vi "testMostCommon.vi"   [LabVIEW 2017]
uses:
  <vilib>/addons/_JKI Toolkits/Caraya/classes/Assert/Assert Equal Value_Variant.vi
  <vilib>/addons/_JKI Toolkits/Caraya/classes/Assert/Assert.lvclass
  <vilib>/addons/_JKI Toolkits/Caraya/classes/Test/Test.lvclass
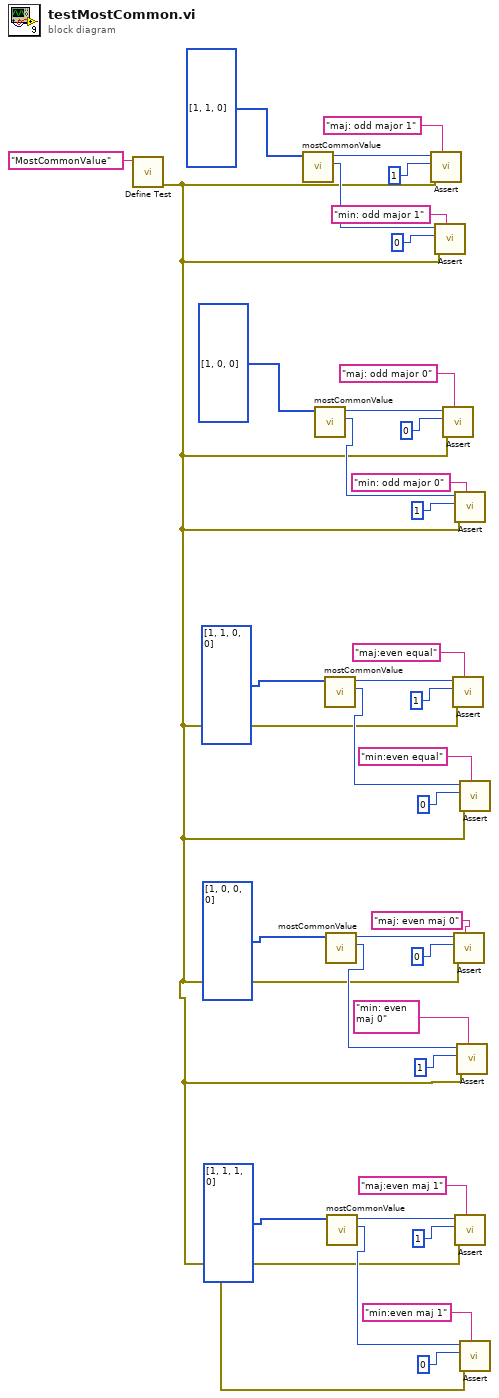
[diagram p0: block diagram]
diagram:
  n1 = call <vilib>:"Define Test.vi"("Label (VI Title)"="MostCommonValue") -> ("error out"=w1:errorcluster)  [unwired: 10 in]
  n2 = call "mostCommonValue.vi"("Array"=i32[] [1, 1, 0]) -> ("Minor"=w16:i32, "Major"=w36:i32)  [unwired: 9 in]
  n3 = call "mostCommonValue.vi"("Array"=i32[] [1, 0, 0]) -> ("Minor"=w11:i32, "Major"=w33:i32)  [unwired: 9 in]
  n4 = call "mostCommonValue.vi"("Array"=i32[] [1, 1, 0, 0]) -> ("Minor"=w8:i32, "Major"=w29:i32)  [unwired: 9 in]
  n5 = call "mostCommonValue.vi"("Array"=i32[] [1, 0, 0, 0]) -> ("Minor"=w2:i32, "Major"=w26:i32)  [unwired: 9 in]
  n6 = call "mostCommonValue.vi"("Array"=i32[] [1, 1, 1, 0]) -> ("Minor"=w3:i32, "Major"=w23:i32)  [unwired: 9 in]
  n7 = call-poly <vilib>:"Assert.vi"("Label"="maj: odd major 1", "error in (no error)"=w1, "Y"=1 ("Numeric"), "X"=w36) -> ()  [unwired: 7 in, 1 out]
  n8 = call-poly <vilib>:"Assert.vi"("Label"="min: odd major 1", "error in (no error)"=w1, "Y"=0 ("Numeric"), "X"=w16) -> ()  [unwired: 7 in, 1 out]
  n9 = call-poly <vilib>:"Assert.vi"("Label"="maj: odd major 0", "error in (no error)"=w1, "Y"=0 ("Numeric"), "X"=w33) -> ()  [unwired: 7 in, 1 out]
  n10 = call-poly <vilib>:"Assert.vi"("Label"="maj:even equal", "error in (no error)"=w1, "Y"=1 ("Numeric"), "X"=w29) -> ()  [unwired: 7 in, 1 out]
  n11 = call-poly <vilib>:"Assert.vi"("Label"="maj: even maj 0", "error in (no error)"=w1, "Y"=0 ("Numeric"), "X"=w26) -> ()  [unwired: 7 in, 1 out]
  n12 = call-poly <vilib>:"Assert.vi"("Label"="min: odd major 0", "error in (no error)"=w1, "Y"=1 ("Numeric"), "X"=w11) -> ()  [unwired: 7 in, 1 out]
  n13 = call-poly <vilib>:"Assert.vi"("Label"="maj:even maj 1", "error in (no error)"=w1, "Y"=1 ("Numeric"), "X"=w23) -> ()  [unwired: 7 in, 1 out]
  n14 = call-poly <vilib>:"Assert.vi"("Label"="min: even maj 0", "error in (no error)"=w1, "Y"=1 ("Numeric"), "X"=w2) -> ()  [unwired: 7 in, 1 out]
  n15 = call-poly <vilib>:"Assert.vi"("Label"="min:even equal", "error in (no error)"=w1, "Y"=0 ("Numeric"), "X"=w8) -> ()  [unwired: 7 in, 1 out]
  n16 = call-poly <vilib>:"Assert.vi"("Label"="min:even maj 1", "error in (no error)"=w1, "Y"=0 ("Numeric"), "X"=w3) -> ()  [unwired: 7 in, 1 out]
